vi "PH_GUI.Manager Minimize.vi"(0 "i ref in":refnum<vi>, 5 "error in":errorcluster) -> (14 "i ref out":refnum<vi>, 19 "error out":errorcluster)   [LabVIEW 2014, in "PH_Common.lvlib"]
doc: "This VI minimizes the GUI of the referenced instnce; this means, the instance is still running while the GUI is removed but accessible by means of the tool bar."
uses:
  PH_Common.lvlib
  CS_Core/CSObj/CSObj.lvlib
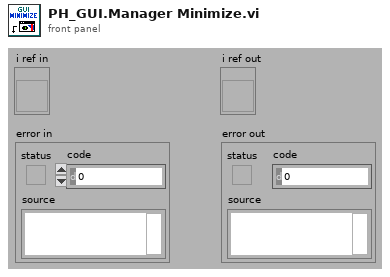
[diagram p1: front panel]
types:
  T1 = enum32{"Invalid", "Standard", "Closed", "Hidden", "Minimized", "Maximized"}
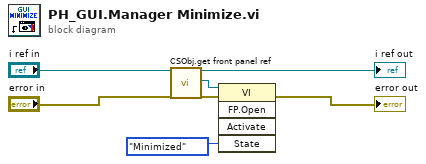
[diagram p0: block diagram]
diagram:
  n1 = call "CSObj.get front panel ref.vi"("i ref in"="i ref in", "error in (no error)"="error in") -> ("i ref out"=→"i ref out":refnum<vi>, "frontPanelRef"=w6:refnum<vi>, "error out"=w4:errorcluster)  [unwired: 15 in]
  n2 = invoke class="VI" method="FP.Open"(reference=w6, error in=w4, "State"=T1."Minimized") -> (error out=→"error out":errorcluster)  [unwired: 2 in, 4 out]
